vi "Create Font by Name and Size.vi"(8 "error in (no error)":errorcluster caption="错误输入（无错误）", 9 "emSize":sgl, 10 "familyName":string) -> (0 "error out":errorcluster caption="错误输出")   [LabVIEW 2011, in "Font.lvclass"]
uses:
  Font.lvclass
  System.Drawing
panel:
  out "new reference":refnum<k24>
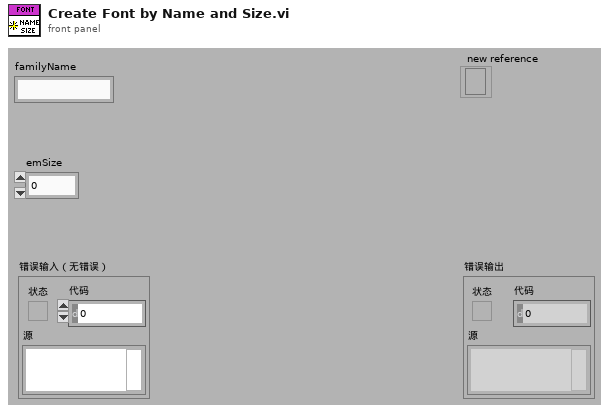
[diagram p1: front panel]
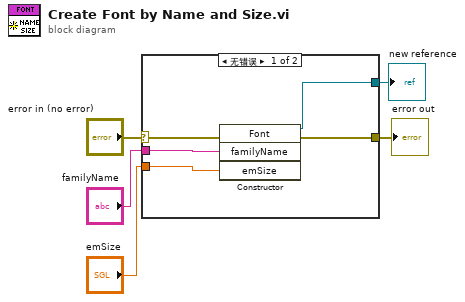
[diagram p0: block diagram]
diagram:
  n1 = case shown="无错误" "error in (no error)" {
    selector: "error in (no error)" -> [w8 w11]
    tunnel: [w7 w11] -> w4
    tunnel: "familyName" -> [w10 _]
    tunnel: "emSize" -> [w9 _]
    tunnel: [w6 _] -> w1
    frame No Error {
      n2 = constructor class="Font"(error in=w8, "familyName"=w10, "emSize"=w9) -> (reference out=w6:refnum<k24>, error out=w7:errorcluster)  [unwired: 2 in, 3 out]
    }
    frame Error {
    }
  }
  "error out" <- w4
  "new reference" <- w1
